vi "Rectangle2miniscans.vi"(10 "Frame Size":i32=200, 11 "X-Y-Z coordinates":T1 {"Z stop" format="%#_6f"; "Z start" format="%#_6f"; "ROI group ID" format="%#_6f"; "Laser Power (%)" format="%#_6f"; "Zoom" format="%#_6f"; "Frame Size" format="%#_6f"; "Number of lines" format="%#_6f"; "Composite ID" format="%#_6f"; "Angle (deg)" format="%#_6f"; "ROI Time (ns)" format="%#_6f"; "ROI ID" format="%#_6f"; "Pixels in ROI" format="%#_6f"; "ROI index" format="%#_6f"; "Y stop" format="%#_6f"; "X stop" format="%#_6f"; "X start" format="%#_6f"; "Y start" format="%#_6f"}) -> (0 "No of Miniscans":i32, 1 "No of Pixels in a single miniscan":i32, 2 "XYZ Stop":cluster{"X":dbl, "Y":dbl, "Z":dbl}[](array[cluster]), 3 "XYZ Start":cluster{"X":dbl, "Y":dbl, "Z":dbl}[](array[cluster]), 4 "Zoom":dbl[](array[numeric]))   [LabVIEW 2017]
uses:
  User Interface/Visualisation/Functional Imaging Viewer/Typedefs/ROI parameters data type.ctl
panel:
  out "miniScan Array":dbl[][](array[numeric])
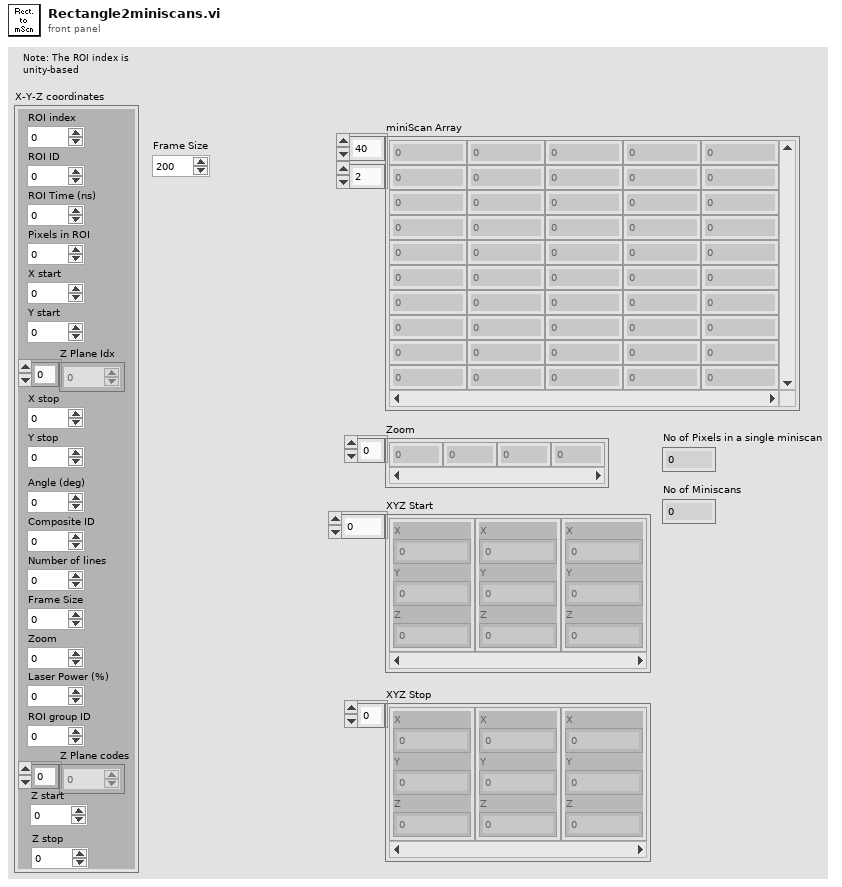
[diagram p1: front panel]
types:
  T1 = typedef "ROI parameters data type.ctl" = cluster{"ROI index":dbl, "ROI ID":dbl, "ROI Time (ns)":dbl, "Pixels in ROI":dbl, "X start":dbl, "Y start":dbl, "X stop":dbl, "Y stop":dbl, "Angle (deg)":dbl, "Composite ID":dbl, "Number of lines":dbl, "Frame Size":dbl, "Zoom":dbl, "Laser Power (%)":dbl, "ROI group ID":dbl, "Z Plane Idx":i32[], "Z Plane codes":u8[], "Z start":dbl, "Z stop":dbl}
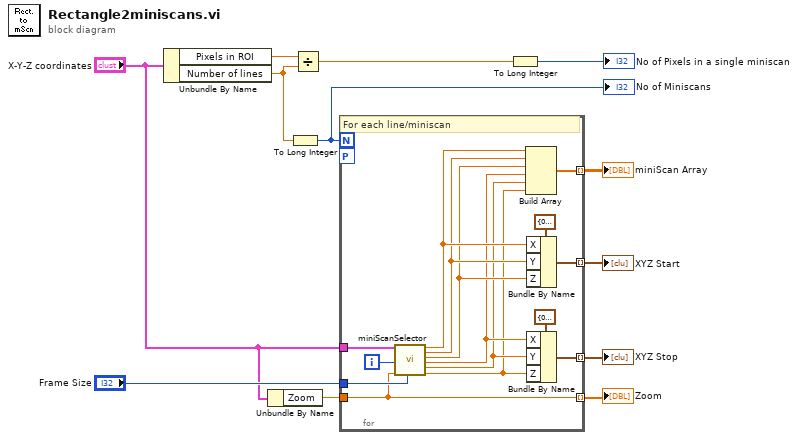
[diagram p0: block diagram]
diagram:
  n1 = Unbundle By Name("X-Y-Z coordinates") -> ("Pixels in ROI"=w5:dbl, "Number of lines"=w8:dbl)
  n2 = Unbundle By Name("X-Y-Z coordinates") -> ("Zoom"=w2:dbl)
  n3 = To Long Integer(number=w8) -> (32bit integer=w6:i32)
  "No of Miniscans" <- w6
  n4 = Divide(x=w5, y=w8) -> (x/y=w3:dbl)
  n5 = for {
    N: w6 -> [_]
    tunnel: [w27] -> w12 mode=indexing
    tunnel: [w26] -> w11 mode=indexing
    tunnel: [w24] -> w10 mode=indexing
    tunnel: "Frame Size" -> [w21]
    tunnel: w2 -> [w13]
    tunnel: [w13] -> w4 mode=indexing
    tunnel: "X-Y-Z coordinates" -> [w22]
    workers-P: _ -> [_]
    i -> [w20]
    # "For each line/miniscan"
    n6 = call "miniScanSelector.vi"("X-Y-Z coordinates"=w22, "index"=w20, "Main zoom"=w13, "FrameSize"=w21) -> ("Norm X Start"=w19:dbl, "Norm Y Start"=w18:dbl, "Norm Z Start"=w17:dbl, "Norm X Stop"=w16:dbl, "Norm Y Stop"=w15:dbl, "Norm Z Stop"=w14:dbl)  [unwired: 10 in]
    n7 = Build Array(w19, w18, w17, w16, w15, w14) -> (w27:dbl[])
    n8 = Bundle By Name(cluster=cluster{"X":dbl, "Y":dbl, "Z":dbl} {"X"=0.0, "Y"=0.0, "Z"=0.0} ("XYZ"), "X"=w19, "Y"=w18, "Z"=w17) -> (w26:cluster{"X":dbl, "Y":dbl, "Z":dbl})
    n9 = Bundle By Name(cluster=cluster{"X":dbl, "Y":dbl, "Z":dbl} {"X"=0.0, "Y"=0.0, "Z"=0.0} ("XYZ"), "X"=w16, "Y"=w15, "Z"=w14) -> (w24:cluster{"X":dbl, "Y":dbl, "Z":dbl})
  }
  "miniScan Array" <- w12
  "XYZ Stop" <- w10
  "XYZ Start" <- w11
  "Zoom" <- w4
  n10 = To Long Integer(number=w3) -> (32bit integer=→"No of Pixels in a single miniscan":i32)
